vi "Read_340-file.vi"() -> ()   [LabVIEW 2018]
uses:
  Instrument_Setup_v2.vi
panel:
  in  "Sensor Name":string
  in  "Nr of calibration data points":dbl=149.0
  out "Original Data":dbl[][](array[numeric]) caption="340 file to Array" format="%#.5g"
  out "xyz.340":string caption="340 file"
  in  "* .340 file path":path=path "D:/CryoTUM_Mischer_Version_2-0/Thermometer/TEST_RuOxTL400_MK_Tail.340"
  # "*.340 file must be prepared beforehand as follows:\n- replace dots with commas: \".\" --> \",\" in data points\n- delimeter in data points must be 1 tab each"
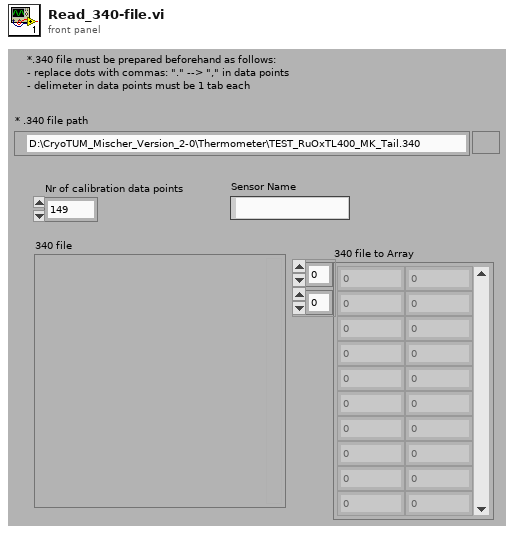
[diagram p1: front panel]
types:
  T1 = enum16{"open", "replace", "create", "open or create", "replace or create", "replace or create with confirmation"}
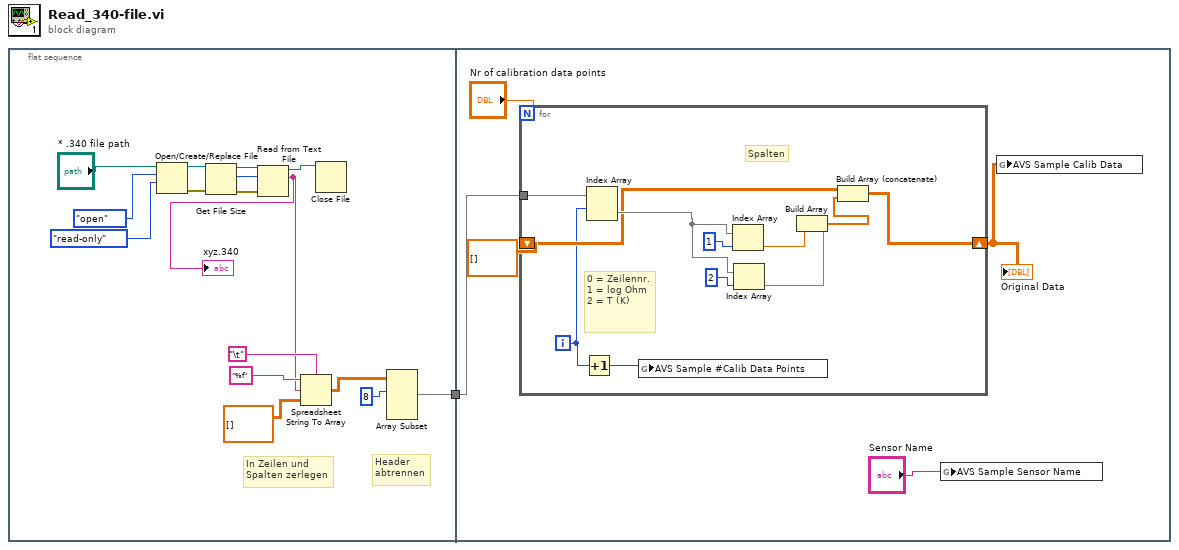
[diagram p0: block diagram]
diagram:
  n1 = flat-sequence {
    tunnel: [w4] -> w1
    tunnel: w1 -> [w22]
    frame #0 {
      # "In Zeilen und \nSpalten zerlegen"
      # "Header\nabtrennen"
      n2 = Open/Create/Replace File(file path (use dialog)="* .340 file path", operation (0:open)=T1."open", access (0:read/write)=enum16{"read/write", "read-only", "write-only"}."read-only") -> (refnum out=w12:refnum<file>, error out=w14:errorcluster)  [unwired: 3 in, 1 out]
      n3 = Get File Size(file=w12, error in=w14) -> (refnum out=w11:refnum<file>, size (in bytes)=w2:i64, 0:w13:errorcluster)
      n4 = Read from Text File(file (use dialog)=w11, count=w2, error in=w13) -> (refnum out=w10:refnum<file>, text=w7:string)  [unwired: 1 in, 2 out]
      "xyz.340" <- w7
      n5 = Spreadsheet String To Array(delimiter (Tab)="\t", format string="%f", spreadsheet string=w7, array type (2D Dbl)=dbl[][] []) -> (array=w3:dbl[][])
      n6 = Close File(refnum=w10) -> ()  [unwired: 1 in, 2 out]
      n7 = Array Subset(array=w3, index (row)=8) -> (w4:dbl[][])  [unwired: 3 in]
    }
    frame #1 {
      n8 = for {
        N: "Nr of calibration data points" -> [_]
        tunnel: w22 -> [w31]
        shift-right: [w26] -> w20
        shift-left: dbl[][] [] -> [w25]
        i -> [w23]
        # "0 = Zeilennr.\n1 = log Ohm\n2 = T (K)"
        # "Spalten"
        n9 = Increment(x=w23) -> (x+1=w24:i32)
        n10 = Index Array(array=w31, index (row)=w23) -> (element=w30:dbl[])  [unwired: 1 in]
        n11 = global write "Instrument_Setup_v2.vi" "AVS Sample #Calib Data Points"(w24) -> ()
        n12 = Index Array(array=w30, index=1) -> (element=w28:dbl)
        n13 = Index Array(array=w30, index=2) -> (element=w29:dbl)
        n14 = Build Array(w28, w29) -> (w27:dbl[])
        n15 = Build Array (concatenate)(w25, w27) -> (w26:dbl[][])
      }
      "Original Data" <- w20
      n16 = global write "Instrument_Setup_v2.vi" "AVS Sample Sensor Name"("Sensor Name") -> ()
      n17 = global write "Instrument_Setup_v2.vi" "AVS Sample Calib Data"(w20) -> ()
    }
  }
